vi "decimal_a_tiempo HOCG.vi"(11 "Numeric 3":dbl) -> (2 "Numeric":dbl, 3 "Numeric 2":dbl format="%#.1g")   [LabVIEW 2021]
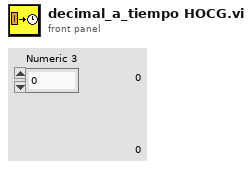
[diagram p1: front panel]
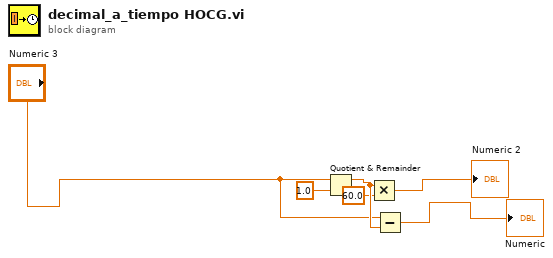
[diagram p0: block diagram]
diagram:
  n1 = Quotient & Remainder(x="Numeric 3", y=1.0) -> (x-y*floor(x/y)=w4:dbl)  [unwired: 1 out]
  n2 = Multiply(x=w4, y=60.0) -> (x*y=→"Numeric 2":dbl)
  n3 = Subtract(x="Numeric 3", y=w4) -> (x-y=→"Numeric":dbl)
